vi "modbus-parameter-to-string.vi"(1 "MODBUS values":u16[](array[numeric]) format="%x") -> (0 "string":string)   [LabVIEW 2015]
doc: "Input: array (length=2) given by Modbus\nThis VI converts\n1 Parameter = 2 Words = 4 Bytes --> 32-bit real\nKeep in mind, that the hexadecimal bytes given by Modbus have to be reversed for conversion!!!"
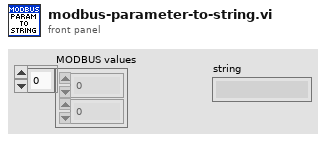
[diagram p1: front panel]
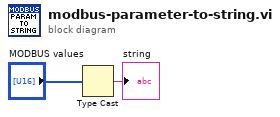
[diagram p0: block diagram]
diagram:
  n1 = Type Cast(x="MODBUS values") -> (*(type *) &x=→"string":string)  [unwired: 1 in]
